vi "Find Library Folder.vi"(7 "Library Name":string, 8 "error in (no error)":errorcluster, 9 "Folder Name":string, 10 "Target Name":string, 11 "Project Sync Tools in":refnum<class "Project Sync Tools.lvclass">) -> (0 "error out":errorcluster, 1 "Found?":bool, 2 "Folder Ref out":refnum<vi>, 3 "Project Sync Tools out":refnum<class "Project Sync Tools.lvclass">)   [LabVIEW 2019, in "Project Sync Tools.lvclass"]
uses:
  Project Sync Tools.lvclass
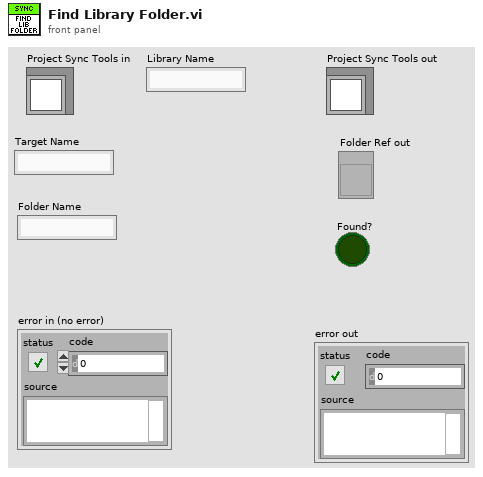
[diagram p1: front panel]
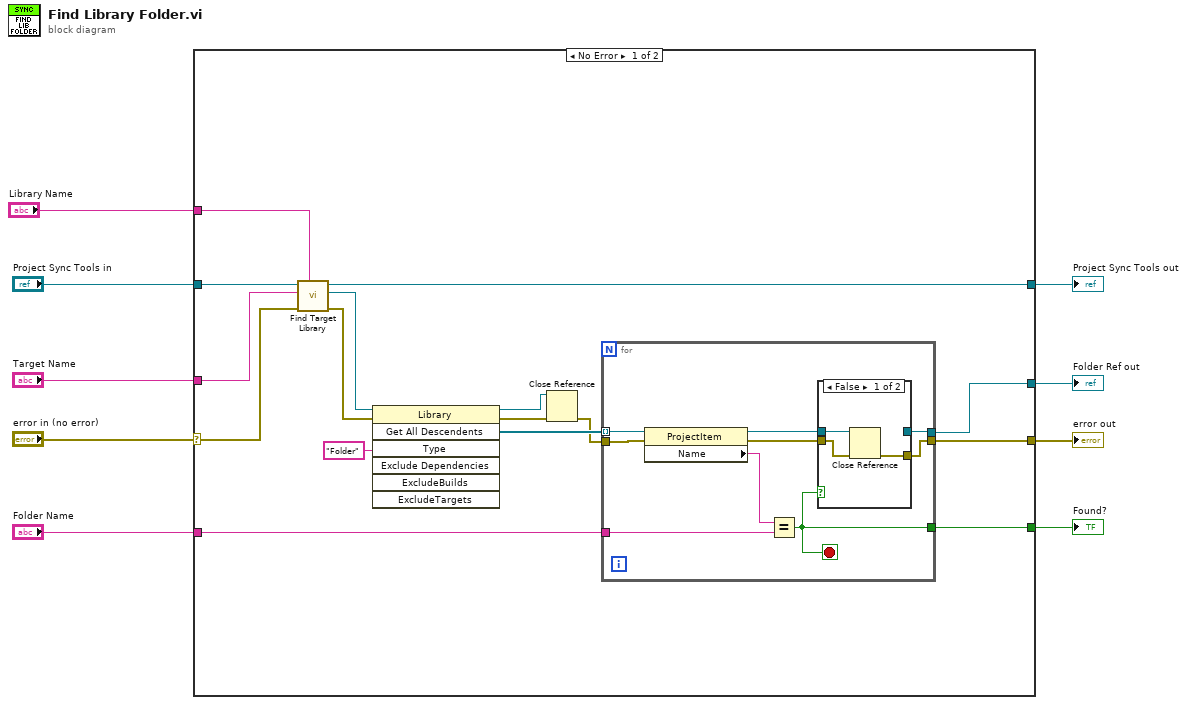
[diagram p0: block diagram]
diagram:
  n1 = case shown="No Error" "error in (no error)" {
    selector: "error in (no error)" -> [w13 w41]
    tunnel: [w25 w41] -> w9
    tunnel: "Folder Name" -> [w24 _]
    tunnel: [w20 w40] -> w7
    tunnel: "Project Sync Tools in" -> [w19 w40]
    tunnel: [w17 _] -> w5
    tunnel: [w16 _] -> w4
    tunnel: "Target Name" -> [w15 _]
    tunnel: "Library Name" -> [w14 _]
    frame No Error {
      n2 = call "Find Target Library.vi"("Library Name"=w14, "error in (no error)"=w13, "Target Name"=w15, "CD Build Tools in"=w19) -> ("error out"=w18:errorcluster, "Library out"=w22:refnum<vi>, "CD Build Tools out"=w20:refnum<class "Project Sync Tools.lvclass">)  [unwired: 4 in, 1 out]
      n3 = invoke class="Library" method="Get All Descendents"(reference=w22, error in=w18, "Type"="Folder") -> (reference out=w11:refnum<vi>, error out=w12:errorcluster, "All Descendents"=w21:refnum<vi>[])  [unwired: 4 in, 4 out]
      n4 = Close Reference(reference=w11, error in (no error)=w12) -> (error out=w10:errorcluster)
      n5 = for {
        tunnel: w21 -> [w34] mode=indexing
        tunnel: w24 -> [w33]
        tunnel: [w28] -> w25
        tunnel: [w31] -> w17
        tunnel: [w27] -> w16
        tunnel: w10 -> [w26]
        stop <- w31 stop-if-true
        n6 = property class="ProjectItem"(reference=w34, error in=w26) -> (reference out=w30:refnum<vi>, error out=w29:errorcluster, "Name"=w32:string)
        n7 = Equal?(x=w32, y=w33) -> (x = y?=w31:bool)
        n8 = case shown="False" w31 {
          tunnel: w30 -> [w37 w39]
          tunnel: w29 -> [w36 w38]
          tunnel: [w35 w38] -> w28
          tunnel: [_ w39] -> w27
          frame False {
            n9 = Close Reference(reference=w37, error in (no error)=w36) -> (error out=w35:errorcluster)
          }
          frame True {
          }
        }
      }
    }
    frame Error {
    }
  }
  "error out" <- w9
  "Project Sync Tools out" <- w7
  "Found?" <- w5
  "Folder Ref out" <- w4
